vi "set gating.vi"(8 "error in (no error)":errorcluster, 10 "Voltage Level":dbl, 11 "VISA resource name":refnum<visa-resource-name>) -> (0 "error out":errorcluster, 3 "VISA resource name out":refnum<visa-resource-name>)   [LabVIEW 2019, in "SubVI.lvlib"]
uses:
  SubVI.lvlib
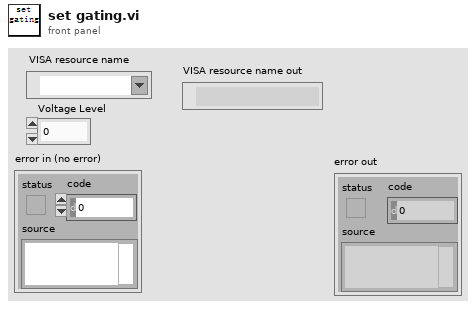
[diagram p1: front panel]
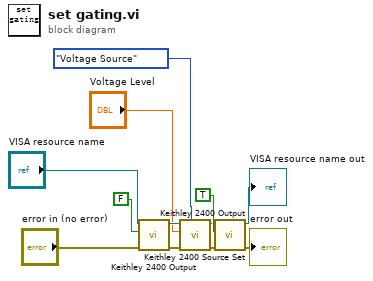
[diagram p0: block diagram]
diagram:
  n1 = call "Keithley 2400 Output.vi"("error in (no error)"="error in (no error)", "Enable Output (T: Enable)"=FALSE, "VISA resource name"="VISA resource name") -> ("error out"=w5:errorcluster, "VISA resource name out"=w8:refnum<visa-resource-name>)  [unwired: 7 in]
  n2 = call "Keithley 2400 Source Set.vi"("Source Type"=enum16{"Voltage Source", "Current Source"}."Voltage Source", "error in (no error)"=w5, "Voltage/curent Level"="Voltage Level", "VISA Refnum in"=w8) -> ("error out"=w4:errorcluster, "VISA Refnum out"=w9:refnum<visa-resource-name>)  [unwired: 6 in]
  n3 = call "Keithley 2400 Output.vi"("error in (no error)"=w4, "Enable Output (T: Enable)"=TRUE, "VISA resource name"=w9) -> ("error out"=→"error out":errorcluster, "VISA resource name out"=→"VISA resource name out":refnum<visa-resource-name>)  [unwired: 7 in]
